vi "_WaitTelemetry.vi"(0 "FIFO":refnum<k21>) -> ()   [LabVIEW 2018, in "Modbus_Processing_Unit.lvlib" / "MPU.lvclass"]
uses:
  MPU.lvclass
  <vilib>/rvi/Emulation/niFpgaGetClockAttributes.vi
  <vilib>/rvi/Emulation/niFpgaSctlEmulationGetInTimedLoop.vi
  <vilib>/rvi/Emulation/niFpgaEmulationReportErrorSimple.vi
  <vilib>/rvi/DataTransferAndStorage/Container/Common/niFpgaContainerExecOnDevCompGetState.vi
  <vilib>/rvi/Emulation/niFpgaEmulationIsFPGAContextNoSignature.vi
  <vilib>/rvi/errors/niFpgaSetErrorForExecOnDevCompSimple.vi
  <vilib>/rvi/eio/common/nirviEmuReportErrorAndStop.vi
  <vilib>/rvi/DataTransferAndStorage/Container/Common/niFpgaContainerGetUniqueNameForEmu.vi
  <vilib>/rvi/FIFO/Fifo_Resource/nirvififoEmulationSetSize.vi
  <vilib>/rvi/FIFO/Fifo_Resource/nirviFifoEmulationQueueMgr.vi
  <instcachedir>/0/nirviFifoEmulationQueueMgr_E5CAEC123FF24DC58D834DCA3CDAA9B5.lvgen/nirviFifoEmulationQueueMgr_E5CAEC123FF24DC58D834DCA3CDAA9B5_001.vi
  <vilib>/rvi/FIFO/Fifo_Resource/nirvififoEmulationDetermineInputValidOut.vi
  <vilib>/rvi/FIFO/Fifo_Resource/nirvififoEmulationCreateLock.vi
  <vilib>/rvi/Emulation/niFpgaProcessEmulError.vi
  <vilib>/rvi/FIFO/Fifo_Resource/nirvififoEmulationObtainLock.vi
  <vilib>/rvi/FIFO/Fifo_Resource/nirvififoEmulationReleaseLock.vi
  <vilib>/rvi/occurrence/nirviWaitOnOccurrenceBase.vi
  <vilib>/rvi/errors/nirviReportUnexpectedCaseInternalError.vi
  <vilib>/rvi/errors/nirviReportUnexpectedCaseInternalError (U32).vi
  <vilib>/Utility/error.llb/Clear Errors.vi
  <vilib>/rvi/interface/RandomDataEmulation/niFpgaRandomDataHandleErrors.vi
  <vilib>/rvi/Emulation/niFpgaCriticalErrorInLSC.vi
  <vilib>/rvi/DataTransferAndStorage/Container/XNode/niFpgaContainer.xnode
  <vilib>/rvi/FIFO/Fifo_Resource/niFpgaFifoEmulationRefIn.vi
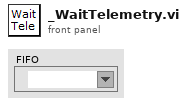
[diagram p1: front panel]
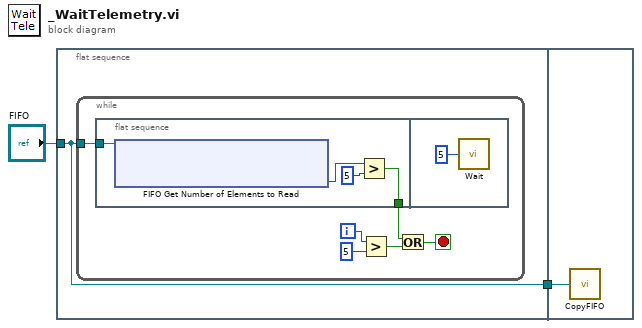
[diagram p0: block diagram]
diagram:
  n1 = flat-sequence {
    tunnel: "FIFO" -> [w3]
    tunnel: [w3] -> w1
    tunnel: w1 -> [w15]
    frame #0 {
      n2 = while {
        tunnel: w3 -> [w4]
        i -> [w7]
        stop <- w8 stop-if-true
        n3 = flat-sequence {
          tunnel: w4 -> [w13]
          tunnel: [w10] -> w9
          frame #0 {
            n4 = xnode "FIFO Get Number of Elements to Read"("FIFO In"=w13) -> ("Number of Elements to Read"=w12:u32)  [unwired: 1 out]
            n5 = Greater?(x=w12, y=u32 5) -> (0:w10:bool)
          }
          frame #1 {
            n6 = call "Wait"("Count(mSec)"=u8 5) -> ()  [unwired: 1 out]
          }
        }
        n7 = Greater?(x=w7, y=5) -> (0:w5:bool)
        n8 = Or(x=w9, y=w5) -> (x .or. y?=w8:bool)
      }
    }
    frame #1 {
      n9 = call "CopyFIFO.vi"("Input"=w15) -> ()
    }
  }
